vi "GetCamera.vi"(3 "error out 2":errorcluster) -> (12 "CCD Chip horizontal end":i32, 14 "CCD Chip Vertical end":i32, 16 "array":i32[][](array[numeric]), 17 "error out":errorcluster, 18 "low":i32, 19 "high":i32, 27 "kinetic":sgl format="%.2f")   [LabVIEW 2013]
uses:
  lib/System Files/user.lib/atmcd32d.llb/ReadMode_mode typedef.ctl
  lib/System Files/user.lib/atmcd32d.llb/AcquisitionMode_mode typedef.ctl
  lib/System Files/user.lib/atmcd32d.llb/TriggerMode_mode typedef.ctl
  lib/System Files/user.lib/atmcd32d.llb/Shutter_type typedef.ctl
  lib/System Files/user.lib/atmcd32d.llb/Shutter_mode typedef.ctl
  lib/System Files/user.lib/atmcd32d.llb/HSSpeed_type typedef.ctl
  lib/System Files/user.lib/atmcd32d.llb/EMGainMode_mode typedef.ctl
  lib/System Files/user.lib/atmcd32d.llb/Error Code Enum typedef.ctl
  GlobalSetGetConfigureCamera.vi
  ccdChipPixels.vi
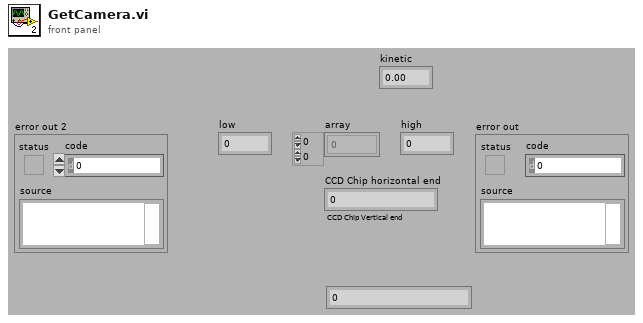
[diagram p1: front panel]
types:
  T1 = typedef "EMGainMode_mode typedef.ctl" = enum16{"8-bit", "12-bit", "Linear", "Real"}
  T2 = typedef "HSSpeed_type typedef.ctl" = enum16{"EM Amp", "Conventional Amp"}
  T3 = typedef "Shutter_mode typedef.ctl" = enum16{"Auto", "Open", "Close"}
  T4 = typedef "Shutter_type typedef.ctl" = enum16{"TTL Low", "TTL High"}
  T5 = typedef "TriggerMode_mode typedef.ctl" = enum16{"Internal", "External", "N/A (2)", "N/A (3)", "N/A (4)", "N/A (5)", "External Start", "External Exposure (Bulb)", "N/A (8)", "External FVB EM", "Software", "N/A (11)", "External Charge Shifting"}
  T6 = typedef "AcquisitionMode_mode typedef.ctl" = enum16{"Reserved (0)", "Single Scan", "Accumulate", "Kinetics", "Fast Kinetics", "Run Till Abort", "Reserved (6)", "Reserved (7)", "Reserved (8)", "Time Delayed Integration"}
  T7 = typedef "ReadMode_mode typedef.ctl" = enum16{"Full Vertical Binning", "Multi-Track", "Random-Track", "Single-Track", "Image"}
  T8 = typedef "Error Code Enum typedef.ctl" = enum32{"N/A (0)", "DRV_ERROR_CODES", "DRV_SUCCESS", "DRV_VXDNOTINSTALLED", "DRV_ERROR_SCAN", "DRV_ERROR_CHECK_SUM", "DRV_ERROR_FILELOAD", "DRV_UNKNOWN_FUNC", "DRV_ERROR_VXD_INIT", "DRV_ERROR_ADDRESS", "DRV_ERROR_PAGELOCK", "DRV_ERROR_PAGEUNLOCK", "DRV_ERROR_BOARDTEST", "DRV_ERROR_ACK", "DRV_ERROR_UP_FIFO", "DRV_ERROR_PATTERN", "N/A (16)", "DRV_ACQUISITION_ERRORS", "DRV_ACQ_BUFFER", "DRV_ACQ_DOWNFIFO_FULL", "DRV_PROC_UNKONWN_INSTRUCTION", "DRV_ILLEGAL_OP_CODE", "DRV_KINETIC_TIME_NOT_MET", "DRV_ACCUM_TIME_NOT_MET", "DRV_NO_NEW_DATA", "N/A (25)", "DRV_SPOOLERROR", "N/A (27)", "N/A (28)", "N/A (29)", "N/A (30)", "N/A (31)", "N/A (32)", "DRV_TEMPERATURE_CODES", "DRV_TEMPERATURE_OFF", "DRV_TEMPERATURE_NOT_STABILIZED", "DRV_TEMPERATURE_STABILIZED", "DRV_TEMPERATURE_NOT_REACHED", "DRV_TEMPERATURE_OUT_RANGE", "DRV_TEMPERATURE_NOT_SUPPORTED", "DRV_TEMPERATURE_DRIFT", "N/A (41)", "N/A (42)", "N/A (43)", "N/A (44)", "N/A (45)", "N/A (46)", "N/A (47)", "N/A (48)", "DRV_GENERAL_ERRORS", "DRV_INVALID_AUX", "DRV_COF_NOTLOADED", "DRV_FPGAPROG", "DRV_FLEXERROR", "DRV_GPIBERROR", "N/A (55)", "N/A (56)", "N/A (57)", "N/A (58)", "N/A (59)", "N/A (60)", "N/A (61)", "N/A (62)", "N/A (63)", "DRV_DATATYPE", "DRV_DRIVER_ERRORS", "DRV_P1INVALID", "DRV_P2INVALID", "DRV_P3INVALID", "DRV_P4INVALID", "DRV_INIERROR", "DRV_COFERROR", "DRV_ACQUIRING", "DRV_IDLE", "DRV_TEMPCYCLE", "DRV_NOT_INITIALIZED", "DRV_P5INVALID", "DRV_P6INVALID", "DRV_INVALID_MODE", "DRV_INVALID_FILTER", "DRV_I2CERRORS", "DRV_I2CDEVNOTFOUND", "DRV_I2CTIMEOUT", "DRV_P7INVALID", "N/A (84)", "N/A (85)", "N/A (86)", "N/A (87)", "N/A (88)", "N/A (89)", "DRV_IOCERROR", "DRV_VRMVERSIONERROR"}
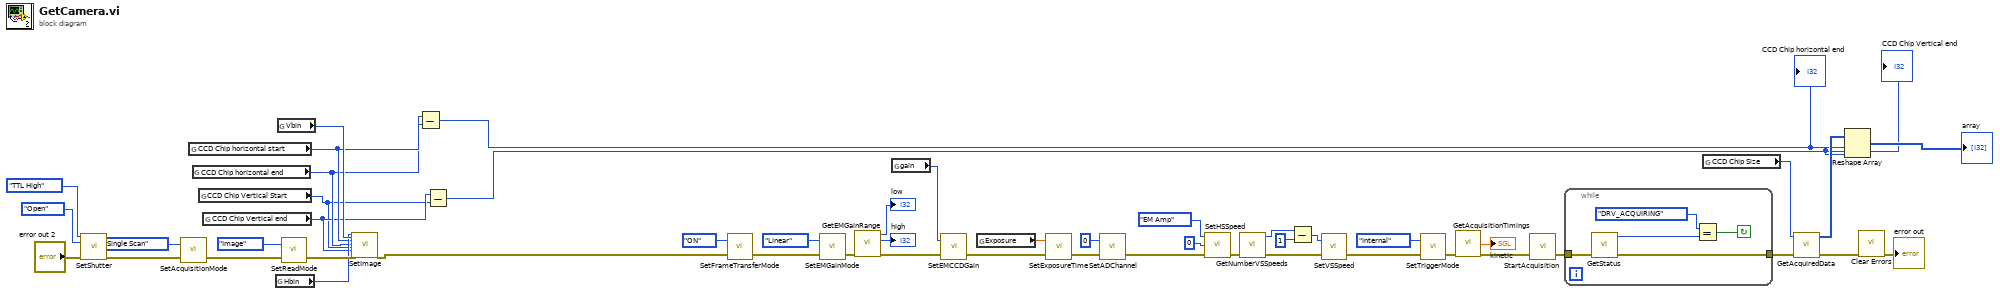
[diagram p0: block diagram]
diagram:
  n1 = call "SetShutter.vi"("type"=Shutter_type_typedef."TTL High", "mode"=Shutter_mode_typedef."Open", "error in (no error)"="error out 2") -> ("error out"=w46:errorcluster)  [unwired: 11 in, 1 out]
  n2 = call "SetAcquisitionMode.vi"("error in (no error)"=w46, "mode"=AcquisitionMode_mode_typedef."Single Scan") -> ("error out"=w22:errorcluster)  [unwired: 1 out]
  n3 = global read "ccdChipPixels.vi" "CCD Chip horizontal start"() -> (w6:i32)
  n4 = global read "ccdChipPixels.vi" "CCD Chip horizontal end"() -> (w5:i32)
  n5 = global read "ccdChipPixels.vi" "CCD Chip Vertical Start"() -> (w1:i32)
  n6 = global read "ccdChipPixels.vi" "CCD Chip Vertical end"() -> (w2:i32)
  n7 = global read "GlobalSetGetConfigureCamera.vi" "Hbin"() -> (w15:i32)
  n8 = global read "GlobalSetGetConfigureCamera.vi" "Vbin"() -> (w16:i32)
  n9 = call "SetReadMode.vi"("error in (no error)"=w22, "mode"=ReadMode_mode_typedef."Image") -> ("error out"=w23:errorcluster)  [unwired: 1 out]
  n10 = call "SetImage.vi"("hbin"=w15, "vbin"=w16, "hstart"=w6, "hend"=w5, "vstart"=w1, "vend"=w2, "error in (no error)"=w23) -> ("error out"=w7:errorcluster)  [unwired: 19 in, 1 out]
  n11 = Subtract(x=w5, y=w6) -> (x-y=w4:i32)
  "CCD Chip horizontal end" <- w4
  n12 = Subtract(x=w2, y=w1) -> (x-y=w3:i32)
  "CCD Chip Vertical end" <- w3
  n13 = call "SetFrameTransferMode.vi"("error in (no error)"=w7, "mode"=enum16{"OFF", "ON"}."ON") -> ("error out"=w17:errorcluster)  [unwired: 1 out]
  n14 = call "SetEMGainMode.vi"("error in (no error)"=w17, "mode"=EMGainMode_mode_typedef."Linear") -> ("error out"=w42:errorcluster)  [unwired: 1 out]
  n15 = call "GetEMGainRange.vi"("error in (no error)"=w42) -> ("error out"=w43:errorcluster, "high"=→"high":i32, "low"=→"low":i32)  [unwired: 3 in, 1 out]
  n16 = global read "GlobalSetGetConfigureCamera.vi" "gain"() -> (w21:i32)
  n17 = call "SetEMCCDGain.vi"("error in (no error)"=w43, "gain"=w21) -> ("error out"=w41:errorcluster)  [unwired: 1 out]
  n18 = global read "GlobalSetGetConfigureCamera.vi" "Exposure"() -> (w20:sgl)
  n19 = call "SetExposureTime.vi"("error in (no error)"=w41, "time"=w20) -> ("error out"=w24:errorcluster)  [unwired: 1 out]
  n20 = call "SetADChannel.vi"("error in (no error)"=w24, "channel"=0) -> ("error out"=w25:errorcluster)  [unwired: 1 out]
  n21 = call "SetHSSpeed.vi"("error in (no error)"=w25, "index"=0, "type"=HSSpeed_type_typedef."EM Amp") -> ("error out"=w29:errorcluster)  [unwired: 1 in, 1 out]
  n22 = call "GetNumberVSSpeeds.vi"("error in (no error)"=w29) -> ("error out"=w31:errorcluster, "number"=w28:i32)  [unwired: 2 in, 1 out]
  n23 = Subtract(x=w28, y=1) -> (x-y=w26:i32)
  n24 = call "SetVSSpeed.vi"("error in (no error)"=w31, "index"=w26) -> ("error out"=w30:errorcluster)  [unwired: 1 out]
  n25 = call "SetTriggerMode.vi"("error in (no error)"=w30, "mode"=TriggerMode_mode_typedef."Internal") -> ("error out"=w11:errorcluster)  [unwired: 1 out]
  n26 = call "GetAcquisitionTimings.vi"("error in (no error)"=w11) -> ("kinetic"=→"kinetic":sgl, "error out"=w10:errorcluster)  [unwired: 10 in, 3 out]
  n27 = call "StartAcquisition.vi"("error in (no error)"=w10) -> ("error out"=w14:errorcluster)  [unwired: 1 in, 1 out]
  n28 = while {
    tunnel: w14 -> [w54]
    tunnel: [w53] -> w13
    stop <- w50 continue-if-true
    n29 = call "GetStatus.vi"("error in (no error)"=w54) -> ("error out"=w53:errorcluster, "status"=w51:T8)  [unwired: 2 in, 1 out]
    n30 = Equal?(x=Error_Code_Enum_typedef."DRV_ACQUIRING" ("status"), y=w51) -> (x = y?=w50:bool)
  }
  n31 = global read "ccdChipPixels.vi" "CCD Chip Size"() -> (w8:i32)
  n32 = call "GetAcquiredData.vi"("error in (no error)"=w13, "size"=w8) -> ("error out"=w12:errorcluster, "array"=w19:i32[])  [unwired: 1 in, 1 out]
  n33 = Reshape Array(w19, w4, w3) -> (→"array":i32[][])
  n34 = call <vilib>:"Clear Errors.vi"("error in (no error)"=w12) -> ("error out"=→"error out":errorcluster)  [unwired: 6 in]
